vi "Temperature and Pressure Monitor.vi"() -> ()   [LabVIEW 2012]
uses:
  <userlib>/_OpenG.lib/numeric/numeric.llb/Random Number Within Range - DBL__ogtk.vi
  <vilib>/addons/database/NI_Database_API.lvlib
panel:
  out "error out":errorcluster
  in  "Graph Time Scales":enum32{"1 Hour (3 sec)", "3 Days (1 Hr)"}(radio)
  out "Temperature (F)":dbl[](graph)
  out "Pressure (torr)":dbl[](graph)
  in  "Stop":bool
  out "Pressure (torr)":dbl
  out "Temperature (F)":dbl
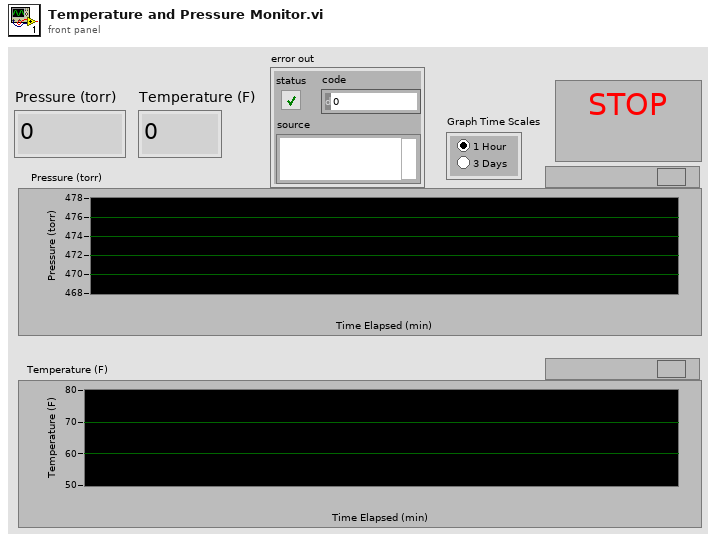
[diagram p1: front panel]
types:
  T1 = typedef "NI_Database_API.lvlib/Conn ObjectReference.ctl" = refnum<k1>
  T2 = cluster{"Integer Time":i64, "Random Number":dbl, dbl}
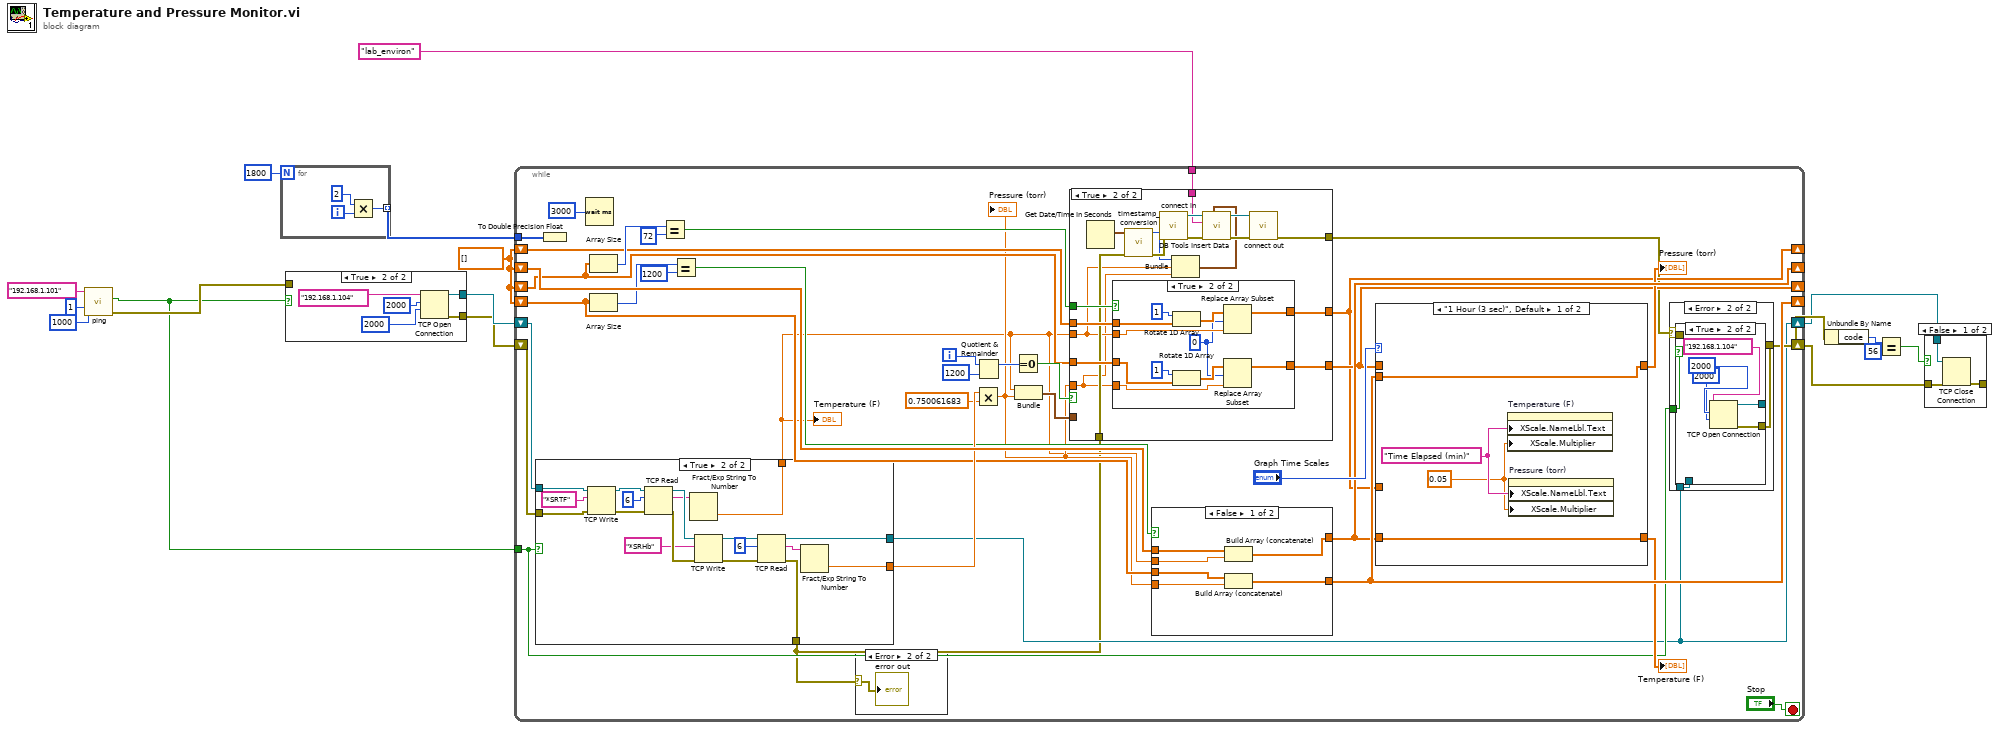
[diagram p0: block diagram]
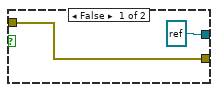
[diagram p2: hidden frame]
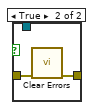
[diagram p3: hidden frame]
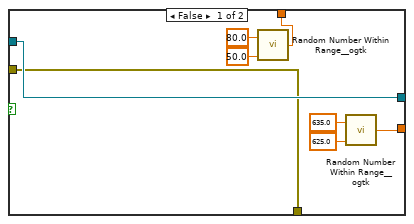
[diagram p7: hidden frame]
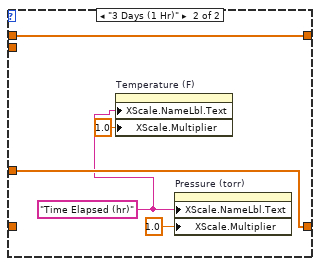
[diagram p8: hidden frame]
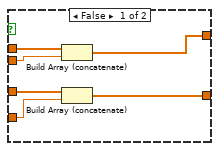
[diagram p10: hidden frame]
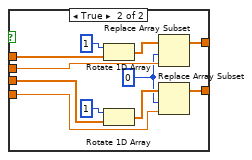
[diagram p11: hidden frame]
diagram:
  w12 = dbl[] []
  n1 = call "ping.vi"("timeout (ms)"=1000, "count"=1, "host"="192.168.1.101") -> ("error out"=w2:errorcluster, "found?"=w1:bool)  [unwired: 6 in, 1 out]
  n2 = for {
    N: 1800 -> [_]
    tunnel: [w17] -> w13 mode=indexing
    i -> [w19]
    n3 = Multiply(x=2, y=w19) -> (x*y=w17:i32)
  }
  n4 = case shown="True" w1 {
    tunnel: [refnum<k5> refnum ("connection ID") w25] -> w16
    tunnel: [w20 w24] -> w15
    tunnel: w2 -> [w20 _]
    frame False {
    }
    frame True {
      n5 = TCP Open Connection(address="192.168.1.104" ("IP Address"), remote port or service name=i16 2000 ("Read Port"), timeout ms (60000)=2000) -> (connection ID=w25:refnum<k5>, error out=w24:errorcluster)  [unwired: 2 in]
    }
  }
  n6 = while {
    shift-right: [w40] -> _
    shift-left: w12 -> [w56]
    shift-right: [w39] -> _
    shift-left: w12 -> [w61]
    tunnel: w13 -> [w59]
    shift-right: [w36] -> _
    shift-left: w12 -> [w44]
    shift-right: [w35] -> _
    shift-left: w12 -> [w43]
    shift-right: [w28] -> w7
    shift-left: w16 -> [w63]
    shift-right: [w31] -> w9
    shift-left: w15 -> [w33]
    tunnel: "lab_environ" ("string") -> [w32]
    tunnel: w1 -> [w29]
    i -> [w52]
    stop <- "Stop" stop-if-true
    n7 = case shown="True" w29 {
      tunnel: w63 -> [w84 w101]
      tunnel: w33 -> [w83 w98]
      tunnel: [w84 w91] -> w28
      tunnel: [w83 w90] -> w27
      tunnel: [w79 w86] -> w60
      tunnel: [w82 w85] -> w34
      frame False {
        n8 = call-poly <userlib>:"Random Number Within Range__ogtk.vi"("High"=80.0, "Low"=50.0) -> ("Random Number"=w82:dbl)  [unwired: 3 in]
        n9 = call-poly <userlib>:"Random Number Within Range__ogtk.vi"("High"=635.0, "Low"=625.0) -> ("Random Number"=w79:dbl)  [unwired: 3 in]
      }
      frame True {
        n10 = TCP Write(connection ID=w101, data in="*SRTF", error in (no error)=w98) -> (connection ID out=w100:refnum<k5>, error out=w97:errorcluster)  [unwired: 1 in, 1 out]
        n11 = TCP Read(connection ID=w100, bytes to read=6, error in (no error)=w97) -> (connection ID out=w93:refnum<k5>, data out=w88:string, error out=w94:errorcluster)  [unwired: 2 in]
        n12 = Fract/Exp String To Number(string=w88) -> (number=w85:dbl)  [unwired: 3 in, 1 out]
        n13 = TCP Write(connection ID=w93, data in="*SRHb", error in (no error)=w94) -> (connection ID out=w95:refnum<k5>, error out=w96:errorcluster)  [unwired: 1 in, 1 out]
        n14 = TCP Read(connection ID=w95, bytes to read=6, error in (no error)=w96) -> (connection ID out=w91:refnum<k5>, data out=w87:string, error out=w90:errorcluster)  [unwired: 2 in]
        n15 = Fract/Exp String To Number(string=w87) -> (number=w86:dbl)  [unwired: 3 in, 1 out]
      }
    }
    "Temperature (F)" <- w34
    n16 = To Double Precision Float(number=w59) -> ()  [unwired: 1 out]
    n17 = Wait (ms)(milliseconds to wait=u32 3000) -> ()  [unwired: 1 out]
    n18 = Array Size(array=w44) -> (size(s)=w47:i32)
    n19 = Array Size(array=w56) -> (size(s)=w55:i32)
    n20 = Equal?(x=w47, y=72) -> (x = y?=w45:bool)
    n21 = Equal?(x=w55, y=1200) -> (x = y?=w53:bool)
    n22 = case shown="Error" w27 {
      selector: w27 -> [_ w64]
      frame No Error {
      }
      frame Error {
        "error out" <- w64
      }
    }
    n23 = Multiply(x=w60, y=0.750061683) -> (x*y=w42:dbl)
    "Pressure (torr)" <- w42
    n24 = Quotient & Remainder(x=w52, y=1200) -> (x-y*floor(x/y)=w50:i32)  [unwired: 1 out]
    n25 = Equal To 0?(x=w50) -> (x = 0?=w49:bool)
    n26 = Bundle("Random Number"=w34, w42) -> (w48:cluster{"Random Number":dbl, dbl})  [unwired: 1 in]
    n27 = case shown="True" w49 {
      tunnel: w48 -> [_ _]
      tunnel: w45 -> [_ w132]
      tunnel: w44 -> [w114 w131]
      tunnel: w43 -> [w113 w130]
      tunnel: w42 -> [_ w116]
      tunnel: w34 -> [_ w117]
      tunnel: [w114 w129] -> w36
      tunnel: [w113 w128] -> w35
      tunnel: w32 -> [_ w125]
      tunnel: w27 -> [w112 w122]
      tunnel: [w112 w119] -> w30
      frame False {
      }
      frame True {
        n28 = Get Date/Time In Seconds() -> (seconds since 1Jan1904=w124:timestamp)
        n29 = case shown="True" w132 {
          tunnel: w131 -> [w138 w149]
          tunnel: w117 -> [w135 w145]
          tunnel: [w134 w142] -> w128
          tunnel: [w136 w141] -> w129
          tunnel: w116 -> [w137 w140]
          tunnel: w130 -> [w133 w139]
          frame False {
            n30 = Build Array (concatenate)(w133, w135) -> (w134:dbl[])
            n31 = Build Array (concatenate)(w138, w137) -> (w136:dbl[])
          }
          frame True {
            w143 = 0 ("index")
            n32 = Rotate 1D Array(1:w139, 2:1 ("n")) -> (0:w146:dbl[])
            n33 = Rotate 1D Array(1:w149, 2:1 ("n")) -> (0:w144:dbl[])
            n34 = Replace Array Subset(array=w146, new element=w145, index=w143) -> (w142:dbl[])
            n35 = Replace Array Subset(array=w144, new element=w140, index=w143) -> (w141:dbl[])
          }
        }
        n36 = call "timestamp_conversion.vi"("error in (no error)"=w122, "Time Stamp"=w124) -> ("error out"=w123:errorcluster, "Integer Time"=w118:i64)  [unwired: 7 in]
        n37 = call "connect in.vi"("error in (no error)"=w123) -> ("error out"=w126:errorcluster, "Database Connection"=w127:T1)  [unwired: 6 in, 1 out]
        n38 = Bundle("Integer Time"=w118, "Random Number"=w117, w116) -> (w115:T2)  [unwired: 1 in]
        n39 = call <vilib>:"DB Tools Insert Data.vi"("data"=w115, "error in (no error)"=w126, "table"=w125, "connection reference"=w127) -> ("error out"=w120:errorcluster, "connection reference out"=w121:T1)  [unwired: 6 in]
        n40 = call "connect out.vi"("error in (no error)"=w120, "connection reference"=w121) -> ("error out"=w119:errorcluster)  [unwired: 9 in]
      }
    }
    n41 = case shown="False" w53 {
      tunnel: w61 -> [w152 w166]
      tunnel: w56 -> [w155 w165]
      tunnel: w34 -> [w151 w161]
      tunnel: [w150 w158] -> w39
      tunnel: [w153 w157] -> w40
      tunnel: w42 -> [w154 w156]
      frame False {
        n42 = Build Array (concatenate)(w152, w151) -> (w150:dbl[])
        n43 = Build Array (concatenate)(w155, w154) -> (w153:dbl[])
      }
      frame True {
        w159 = 0 ("index")
        n44 = Rotate 1D Array(1:w166, 2:1 ("n")) -> (0:w162:dbl[])
        n45 = Rotate 1D Array(1:w165, 2:1 ("n")) -> (0:w160:dbl[])
        n46 = Replace Array Subset(array=w162, new element=w161, index=w159) -> (w158:dbl[])
        n47 = Replace Array Subset(array=w160, new element=w156, index=w159) -> (w157:dbl[])
      }
    }
    n48 = case shown="\"1 Hour (3 sec)\", Default" "Graph Time Scales" {
      tunnel: w40 -> [w105 _]
      tunnel: w39 -> [w106 _]
      tunnel: [w106 w110] -> w38
      tunnel: [w105 w111] -> w37
      tunnel: w36 -> [_ w111]
      tunnel: w35 -> [_ w110]
      frame "1 Hour (3 sec)", Default {
        w103 = 0.05 ("X Scale.Offset and Multiplier:Multiplier")
        w104 = "Time Elapsed (min)" ("Y Scale.Name Label.Text")
        n49 = property on="Temperature (F)" class="WFGraph (strict)"("XScale.NameLbl.Text"=w104, "XScale.Multiplier"=w103) -> ()  [unwired: 2 in, 2 out]
        n50 = property on="Pressure (torr)" class="WFGraph (strict)"("XScale.NameLbl.Text"=w104, "XScale.Multiplier"=w103) -> ()  [unwired: 2 in, 2 out]
      }
      frame "3 Days (1 Hr)" {
        w107 = "Time Elapsed (hr)" ("Y Scale.Name Label.Text")
        n51 = property on="Temperature (F)" class="WFGraph (strict)"("XScale.NameLbl.Text"=w107, "XScale.Multiplier"=1.0 ("Y Scale.Offset and Multiplier:Multiplier")) -> ()  [unwired: 2 in, 2 out]
        n52 = property on="Pressure (torr)" class="WFGraph (strict)"("XScale.NameLbl.Text"=w107, "XScale.Multiplier"=1.0 ("X Scale.Offset and Multiplier:Multiplier")) -> ()  [unwired: 2 in, 2 out]
      }
    }
    "Pressure (torr)" <- w37
    "Temperature (F)" <- w38
    n53 = case shown="Error" w30 {
      selector: w30 -> [w65 w69]
      tunnel: [w65 w68] -> w31
      tunnel: w29 -> [_ w66]
      tunnel: w28 -> [_ w67]
      frame No Error {
      }
      frame Error {
        n54 = case shown="True" w66 {
          tunnel: [w70 w75] -> _
          tunnel: [w71 w74] -> w68
          tunnel: w69 -> [w71 _]
          tunnel: w67 -> [w70 _]
          frame False {
          }
          frame True {
            n55 = TCP Open Connection(address="192.168.1.104" ("IP Address"), remote port or service name=i16 2000 ("Read Port"), timeout ms (60000)=2000) -> (connection ID=w75:refnum<k5>, error out=w74:errorcluster)  [unwired: 2 in]
          }
        }
      }
    }
  }
  n56 = Unbundle By Name(w9) -> ("code"=w11:i32)
  n57 = Equal?(x=w11, y=56) -> (x = y?=w8:bool)
  n58 = case shown="False" w8 {
    tunnel: w9 -> [w169 w171]
    tunnel: [w168 w170] -> _
    tunnel: w7 -> [w167 _]
    frame False {
      n59 = TCP Close Connection(connection ID=w167, error in (no error)=w169) -> (error out=w168:errorcluster)  [unwired: 1 in, 1 out]
    }
    frame True {
      n60 = call <vilib>:"Clear Errors.vi"("error in (no error)"=w171) -> ("error out"=w170:errorcluster)  [unwired: 6 in]
    }
  }
